vi "PQclear.vi"(8 "error in (no error)":errorcluster, 10 "res":u64, 11 "conn":u64) -> (0 "error out":errorcluster, 3 "conn_out":u64)   [LabVIEW 2019, in "libpqlv64.lvlib"]
doc: "Frees the storage associated with a PGresult. Every command result should be freed via PQclear when it is no longer needed.\n\nYou can keep a PGresult object around for as long as you need it; it does not go away when you issue a new command, nor even if you close the connection. To get rid of it, you must call PQclear. Failure to do this will result in memory leaks in your application."
uses:
  libpqlv64.lvlib
  libpq.dll
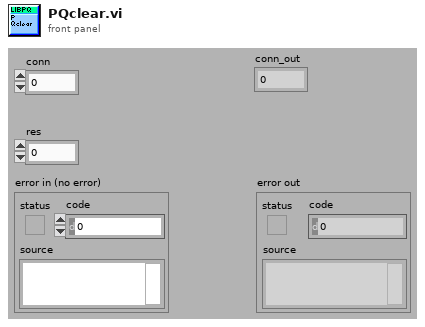
[diagram p1: front panel]
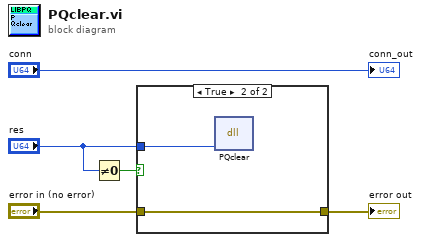
[diagram p0: block diagram]
diagram:
  n1 = Not Equal To 0?(x="res") -> (x != 0?=w4:bool)
  n2 = case shown="True" w4 {
    tunnel: "res" -> [_ w8]
    tunnel: "error in (no error)" -> [w6 w7]
    tunnel: [w6 w7] -> w1
    frame False {
    }
    frame True {
      n3 = dll-call lib="libpq.*" fn="PQclear"("res"=w8) -> ()  [unwired: 5 in, 2 out]
    }
  }
  "error out" <- w1
  "conn_out" <- "conn"
